vi "Calculator_multiply-setup.vi"(8 "test case ID":string) -> (1 "b":dbl, 2 "a":dbl, 3 "Calculator in":refnum<class "Calculator.lvclass">)   [LabVIEW 2018]
doc: "The setup VI should be executed before the VI under test in the harness VI. In this VI you can prepare the environment and the inputs of the VI under test.\n\nSee the Help Document for more information. (<b>Help</b> > <b>InstaCoverage Help...</b>)"
uses:
  Calculator.lvclass
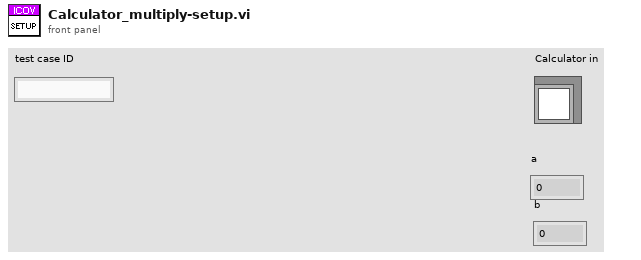
[diagram p1: front panel]
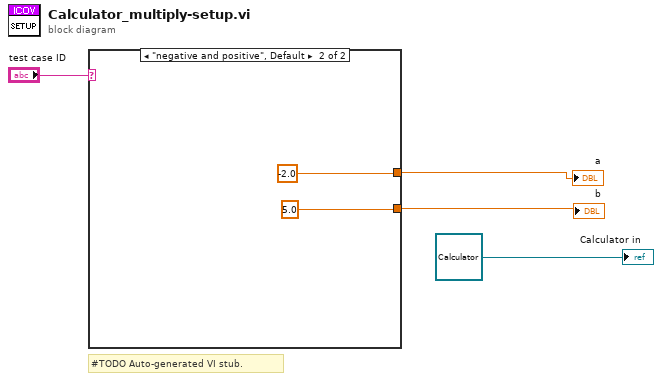
[diagram p0: block diagram]
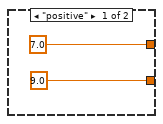
[diagram p2: hidden frame]
diagram:
  # "#TODO Auto-generated VI stub."
  n1 = case shown="\"negative and positive\", Default" "test case ID" {
    tunnel: [7.0 ("a") -2.0 ("a")] -> w1
    tunnel: [9.0 ("a") 5.0 ("a")] -> w3
    frame "positive" {
    }
    frame "negative and positive", Default {
    }
  }
  "a" <- w1
  "b" <- w3
  "Calculator in" <- refnum<class "Calculator.lvclass"> refnum ("Calculator in")
